vi "claseparte3_13_01_2021.vi"() -> ()   [LabVIEW 2020]
panel:
  in  "Time Target (s)":dbl=30.0
  in  "stop":bool
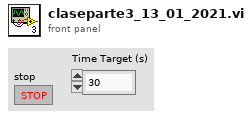
[diagram p1: front panel]
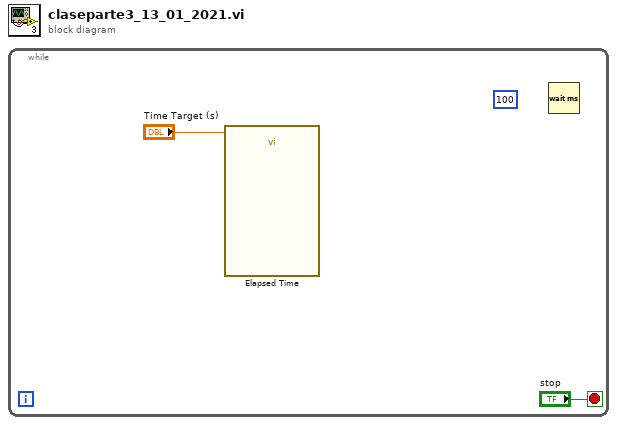
[diagram p0: block diagram]
diagram:
  n1 = while {
    stop <- "stop" stop-if-true
    (unwired) 100
    n2 = call "Elapsed Time"("Time Target (s)"="Time Target (s)") -> ()  [unwired: 11 in, 8 out]
    n3 = Wait (ms)() -> ()  [unwired: 1 in, 1 out]
  }
